vi "Configure (Port and DB).vi"(8 "error in (no error)":errorcluster, 11 "Device Item Ref in":T1 format="%.0x") -> (0 "error out":errorcluster, 3 "Device Item Ref out":T1 format="%.0x")   [LabVIEW 2020, in "FlexRay Custom Device System Explorer.lvlib"]
uses:
  FlexRay Custom Device System Explorer.lvlib
  Shared/FRInterface.ctl
  <vilib>/NI VeriStand/Custom Device API/Custom Device Item Ref.ctl
  Shared/FRConfig.ctl
  Shared/Constants.vi
  <vilib>/NI VeriStand/Custom Device API/Set Item Property (Variant).vi
  <vilib>/Utility/error.llb/Error Cluster From Error Code.vi
  <vilib>/ErrorRing/Error Ring.xnode
  <resource>/objmgr/xnet.rc
  <vilib>/NI VeriStand/Custom Device API/Custom Device API.lvlib
  Shared/FlexRay Custom Device Shared.lvlib
panel:
  in  "Cancel":bool
  in  "OK":bool
  in  "FlexRay Cluster":u16(ring) items=["FlexRay_Cluster"]
  in  "FlexRay Interface":T2 items=["FlexRay1", "FlexRay2", "FlexRay3", "FlexRay4", "FlexRay5", "FlexRay6", "FlexRay7", "FlexRay8"]
  in  "XNET Database":refnum<k21>
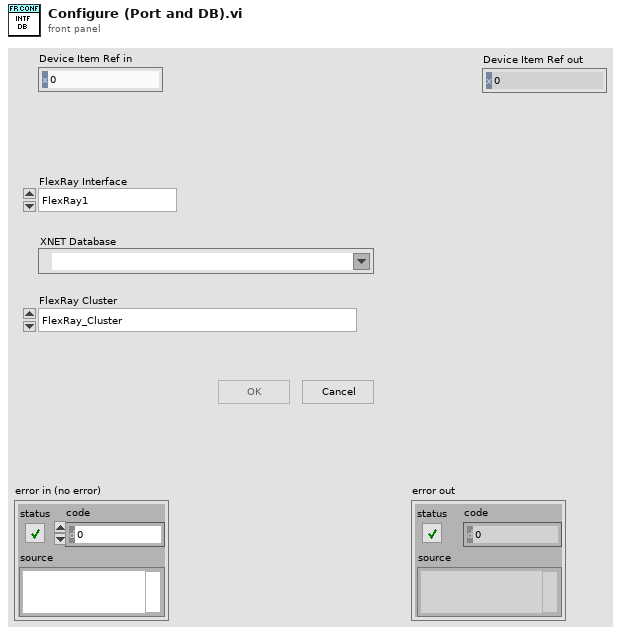
[diagram p1: front panel]
types:
  T1 = typedef "Custom Device API.lvlib/Custom Device Item Ref.ctl" = u64
  T2 = typedef "FlexRay Custom Device Shared.lvlib/FRInterface.ctl" = u16
  T3 = typedef "FlexRay Custom Device Shared.lvlib/FRConfig.ctl" = cluster{"FlexRay Interface":T2, "XNET Database":refnum<k21>, "XNET Cluster":refnum<k21>, "ColdStart ID":u32, "Termination":bool}
  T4 = cluster{"Availble XNET Clusters":refnum<k21>[], "FRConfig":T3}
  T5 = enum8{"Enabled", "Disabled", "Disabled and Grayed Out"}
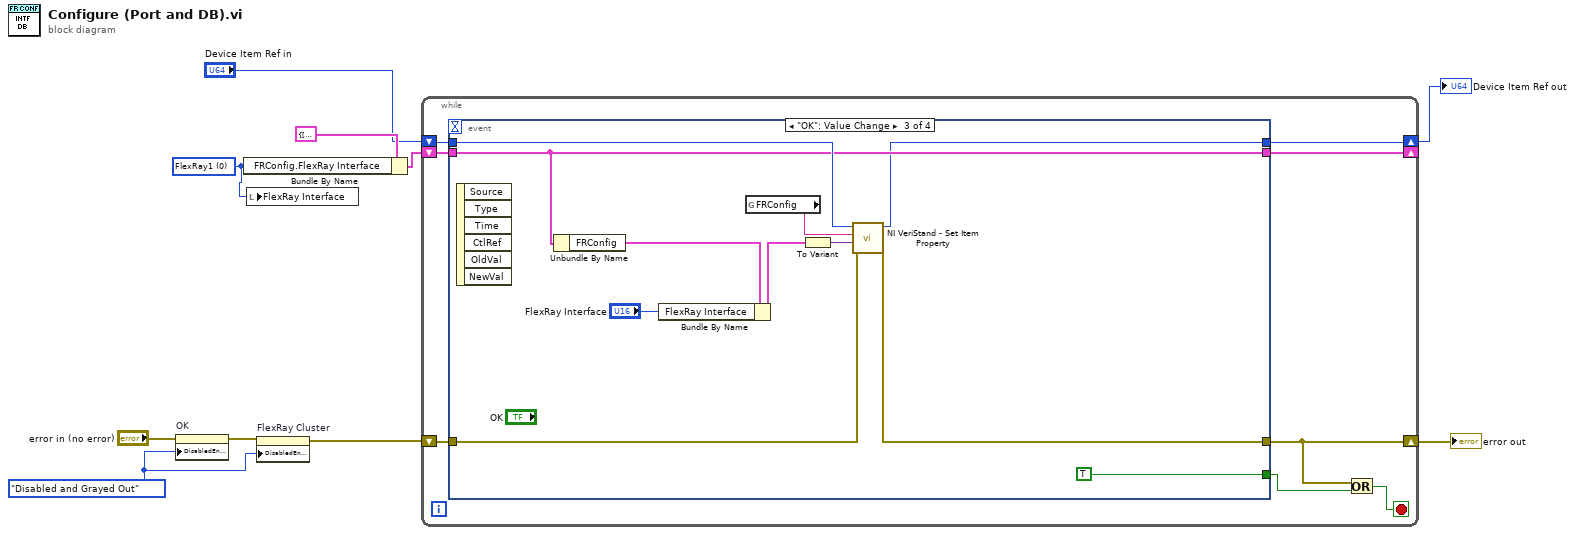
[diagram p0: block diagram]
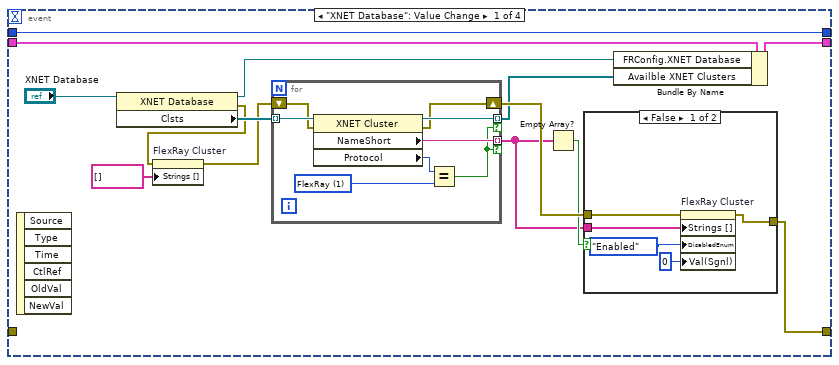
[diagram p2: hidden frame]
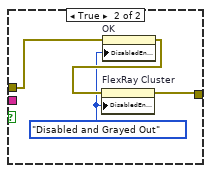
[diagram p3: hidden frame]
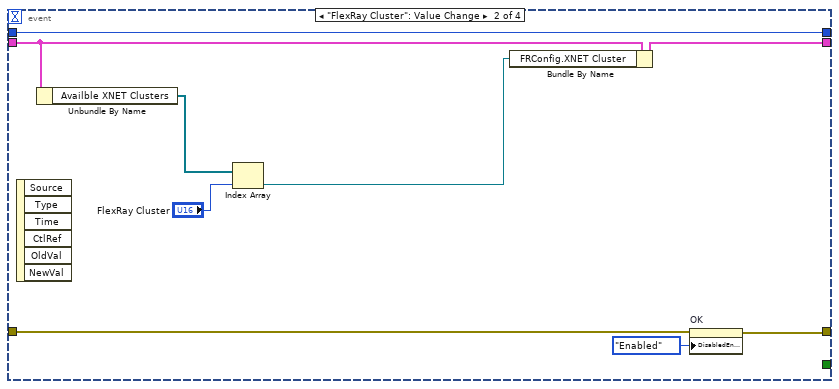
[diagram p4: hidden frame]
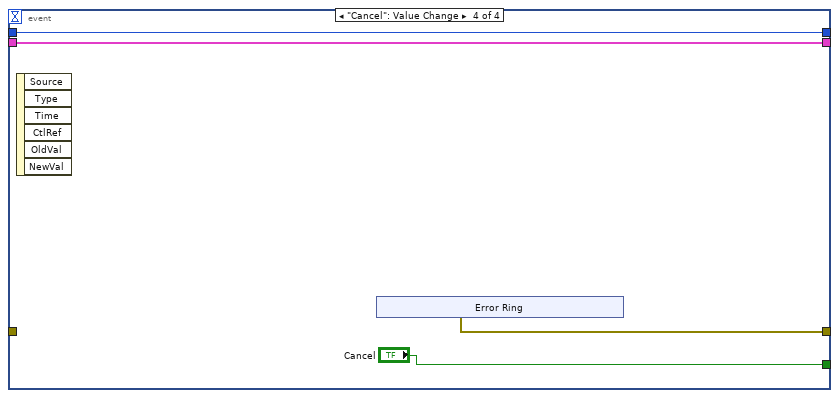
[diagram p5: hidden frame]
diagram:
  w1 = T2 0 items=["FlexRay1", "FlexRay2", "FlexRay3", "FlexRay4", "FlexRay5", "FlexRay6", "FlexRay7", "FlexRay8"] ("FlexRay Interface")
  w6 = T5."Disabled and Grayed Out" ("Disabled")
  n1 = property on="OK" class="Bool"(error in="error in (no error)", "DisabledEnum"=w6) -> (error out=w8:errorcluster)  [unwired: 1 in, 1 out]
  n2 = Bundle By Name(cluster=T4 {"Availble XNET Clusters"=[], "FRConfig"={"FlexRay Interface"=0, "XNET Database"="", "XNET Cluster"="", "ColdStart ID"=0, "Termination"=FALSE}}, "FRConfig.FlexRay Interface"=w1) -> (w4:T4)
  n3 = local write "FlexRay Interface"(w1) -> ()
  n4 = property on="FlexRay Cluster" class="Ring (strict)"(error in=w8, "DisabledEnum"=w6) -> (error out=w7:errorcluster)  [unwired: 1 in, 1 out]
  n5 = while {
    shift-right: [w17] -> w10
    shift-left: w7 -> [w18]
    shift-right: [w13] -> _
    shift-left: w4 -> [w14]
    shift-right: [w11] -> w3
    shift-left: "Device Item Ref in" -> [w12]
    stop <- w16 stop-if-true
    n6 = event shown="[2] \"OK\": Value Change" {
      selector: _ -> [_ _ _ _]
      dyn-events: _ -> [_ _ _ _]
      timeout: _ -> [_ _ _ _]
      tunnel: w18 -> [_ w53 w65 _]
      tunnel: [w20 w54 w64 w72] -> w17
      tunnel: [_ _ TRUE ("Cancel") "Cancel"] -> w15
      tunnel: w14 -> [w24 w56 w63 w70]
      tunnel: [w23 w58 w63 w70] -> w13
      tunnel: w12 -> [w19 w51 w66 w71]
      tunnel: [w19 w51 w61 w71] -> w11
      event "XNET Database": Value Change {
        n7 = event-data() -> ()  [unwired: 1 in, 6 out]
        n8 = property class="XNET Database"(reference="XNET Database") -> (reference out=w22:refnum<k21>, error out=w29:errorcluster, "Clsts"=w32:refnum<k21>[])  [unwired: 1 in]
        n9 = property on="FlexRay Cluster" class="Ring (strict)"(error in=w29, "Strings []"=string[] []) -> (error out=w28:errorcluster)  [unwired: 1 in, 1 out]
        n10 = for {
          tunnel: w32 -> [w49] mode=indexing
          tunnel: [w48] -> w25 mode=indexing if=w44
          tunnel: [w45] -> w21 mode=indexing if=w44
          shift-right: [w42] -> w27
          shift-left: w28 -> [w43]
          w46 = u32 1 items=["CAN", "FlexRay", "LIN"] ("Protocol")
          n11 = property class="XNET Cluster"(reference=w49, error in=w43) -> (reference out=w45:refnum<k21>, error out=w42:errorcluster, "NameShort"=w48:string, "Protocol"=w47:u32)
          n12 = Equal?(x=w47, y=w46) -> (x = y?=w44:bool)
        }
        n13 = Empty Array?(array=w25) -> (empty?=w26:bool)
        n14 = case shown="False" w26 {
          tunnel: w25 -> [w37 _]
          tunnel: w27 -> [w36 w41]
          tunnel: [w33 w38] -> w20
          frame False {
            n15 = property on="FlexRay Cluster" class="Ring (strict)"(error in=w36, "Strings []"=w37, "DisabledEnum"=T5."Enabled" ("Disabled"), "Val(Sgnl)"=u16 0 ("Value (Signaling)")) -> (error out=w33:errorcluster)  [unwired: 1 in, 1 out]
          }
          frame True {
            w39 = T5."Disabled and Grayed Out" ("Disabled")
            n16 = property on="OK" class="Bool"(error in=w41, "DisabledEnum"=w39) -> (error out=w40:errorcluster)  [unwired: 1 in, 1 out]
            n17 = property on="FlexRay Cluster" class="Ring (strict)"(error in=w40, "DisabledEnum"=w39) -> (error out=w38:errorcluster)  [unwired: 1 in, 1 out]
          }
        }
        n18 = Bundle By Name(cluster=w24, "FRConfig.XNET Database"=w22, "Availble XNET Clusters"=w21) -> (w23:T4)
      }
      event "FlexRay Cluster": Value Change {
        n19 = event-data() -> ()  [unwired: 1 in, 6 out]
        n20 = Unbundle By Name(w56) -> ("Availble XNET Clusters"=w55:refnum<k21>[])
        n21 = Index Array(array=w55, index="FlexRay Cluster") -> (element=w50:refnum<k21>)
        n22 = Bundle By Name(cluster=w56, "FRConfig.XNET Cluster"=w50) -> (w58:T4)
        n23 = property on="OK" class="Bool"(error in=w53, "DisabledEnum"=T5."Enabled" ("Disabled")) -> (error out=w54:errorcluster)  [unwired: 1 in, 1 out]
      }
      event "OK": Value Change {
        n24 = event-data() -> ()  [unwired: 1 in, 6 out]
        n25 = Unbundle By Name(w63) -> ("FRConfig"=w68:T3)
        n26 = Bundle By Name(cluster=w68, "FlexRay Interface"="FlexRay Interface") -> (w60:T3)
        n27 = global read "Constants.vi" "FRConfig"() -> (w62:string)
        n28 = To Variant(anything=w60) -> (Variant=w67:variant)
        n29 = call-poly <vilib>:"NI VeriStand - Set Item Property.vi"("error in (no error)"=w65, "Value"=w67, "Property Name"=w62, "Item Ref in"=w66) -> ("error out"=w64:errorcluster, "Item Ref out"=w61:T1)  [unwired: 5 in, 1 out]
      }
      event "Cancel": Value Change {
        n30 = event-data() -> ()  [unwired: 1 in, 6 out]
        n31 = xnode "Error Ring"() -> ("error out"=w72:errorcluster)
      }
    }
    n32 = Or(x=w17, y=w15) -> (x .or. y?=w16:bool)
  }
  "Device Item Ref out" <- w3
  "error out" <- w10
